vi "AskForConnectedSCDs.vi"(7 "DiscoverDevices in":T1, 8 "error in (no error)":errorcluster, 9 "delimiter of string answer (semicolon)":string=";", 10 "timeout for receiving data [ms]":i32=5000, 11 "Communicator in":refnum<class "Communicator.lvclass">) -> (0 "error out":errorcluster, 2 "DiscoverDevices out":T1, 3 "Communicator out":refnum<class "Communicator.lvclass">, 5 "unformated list of devices":string[](array[string]))   [LabVIEW 2023, in "DeviceManager.lvlib"]
uses:
  DeviceManager.lvlib
  DiscoverDevices (Reply Payload)--cluster.ctl
  Classes/Mono/Monochromator.lvclass
  Classes/CCD/CCD.lvclass
  Classes/SCD/SCD.lvclass
  Classes/Communicator/Communicator.lvclass
panel:
  # "Connector Pane"
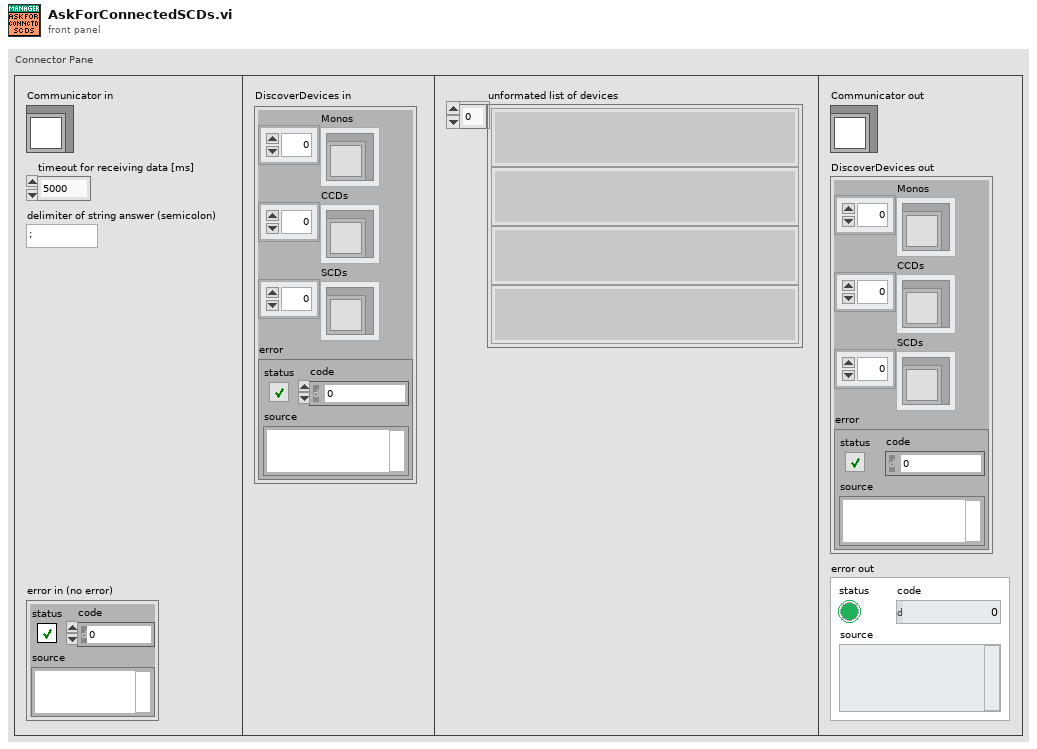
[diagram p1: front panel]
types:
  T1 = typedef "DeviceManager.lvlib/DiscoverDevices (Reply Payload)--cluster.ctl" = cluster{"Monos":refnum<class "Monochromator.lvclass">[], "CCDs":refnum<class "CCD.lvclass">[], "SCDs":refnum<class "SCD.lvclass">[], "error":errorcluster}
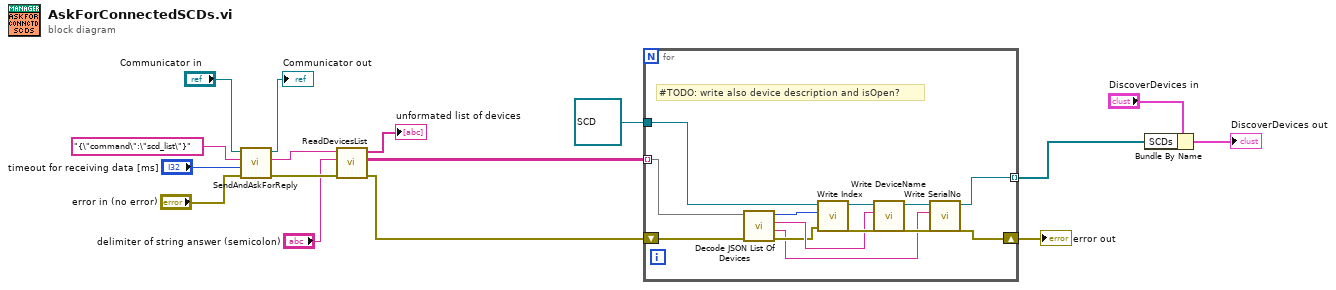
[diagram p0: block diagram]
diagram:
  n1 = call-dynamic "SendAndAskForReply.vi"("error in (no error)"="error in (no error)", "timeout for receiving data [ms]"="timeout for receiving data [ms]", "String to be sent"="{\"command\":\"scd_list\"}", "Communicator in"="Communicator in") -> ("error out"=w12:errorcluster, "Data"=w11:string, "Communicator out"=→"Communicator out":refnum<class "Communicator.lvclass">)  [unwired: 5 in]
  n2 = call "ReadDevicesList.vi"("error in"=w12, "delimiter of string answer (semicolon)"="delimiter of string answer (semicolon)", "JSON"=w11) -> ("error out"=w14:errorcluster, "table of devices"=w15:string[][], "unformated list of devices"=→"unformated list of devices":string[])  [unwired: 6 in]
  n3 = for {
    tunnel: w15 -> [w26] mode=indexing
    shift-right: [w21] -> w3
    shift-left: w14 -> [w27]
    tunnel: [w19] -> w5 mode=indexing
    tunnel: refnum<class "SCD.lvclass"> refnum ("SCD.lvclass") -> [w22]
    # "#TODO: write also device description and isOpen?"
    n4 = call "Decode JSON List Of Devices.vi"("error in"=w27, "table of devices"=w26) -> ("error out"=w23:errorcluster, "description with Serial Number"=w17:string, "name of device"=w24:string, "device index"=w25:i32)  [unwired: 6 in]
    n5 = call-dynamic "Write Index.vi"("error in (no error)"=w23, "Index"=w25, "SCD in"=w22) -> ("error out"=w28:errorcluster, "SCD out"=w29:refnum<class "SCD.lvclass">)  [unwired: 7 in]
    n6 = call-dynamic "Write DeviceName.vi"("error in (no error)"=w28, "DeviceName"=w24, "SCD in"=w29) -> ("error out"=w20:errorcluster, "SCD out"=w18:refnum<class "SCD.lvclass">)  [unwired: 7 in]
    n7 = call-dynamic "Write SerialNo.vi"("error in (no error)"=w20, "SerialNo"=w17, "SCD in"=w18) -> ("error out"=w21:errorcluster, "SCD out"=w19:refnum<class "SCD.lvclass">)  [unwired: 7 in]
  }
  "error out" <- w3
  n8 = Bundle By Name(cluster="DiscoverDevices in", "SCDs"=w5) -> (→"DiscoverDevices out":T1)
